vi "7.vi"() -> ()   [LabVIEW 2017, in "ErrorStructureDrawer-Tests.lvlib"]
uses:
  ErrorStructureDrawer-Tests.lvlib
panel:
  out "path":path
  in  "file path (use dialog)":path
  in  "operation (0:open)":T1(ring)
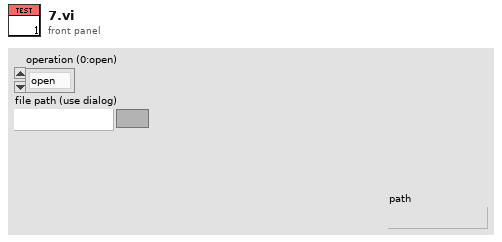
[diagram p1: front panel]
types:
  T1 = enum16{"open", "replace", "create", "open or create", "replace or create", "replace or create with confirmation"}
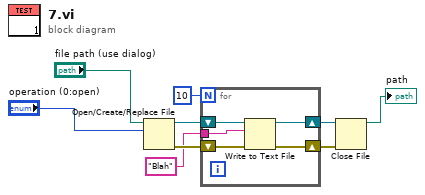
[diagram p0: block diagram]
diagram:
  n1 = Open/Create/Replace File(file path (use dialog)="file path (use dialog)", operation (0:open)="operation (0:open)") -> (refnum out=w9:refnum<file>, error out=w7:errorcluster)  [unwired: 4 in, 1 out]
  n2 = for {
    N: 10 -> [_]
    shift-right: [w13] -> w8
    shift-left: w9 -> [w14]
    shift-right: [w11] -> w6
    shift-left: w7 -> [w12]
    tunnel: "Blah" -> [w10]
    n3 = Write to Text File(file (use dialog)=w14, text=w10, error in=w12) -> (refnum out=w13:refnum<file>, error out=w11:errorcluster)  [unwired: 1 in, 1 out]
  }
  n4 = Close File(refnum=w8, error in=w6) -> (path=→"path":path)  [unwired: 1 out]
